vi "Initialize-object.vi"(7 "Heartbeat interval":dbl, 8 "error in (no error)":errorcluster, 9 "Client channel":refnum<queue>, 10 "Server channel":refnum<queue>) -> (0 "error out":errorcluster, 3 "Reference out":T1)   [LabVIEW 2013, in "CameraVision.lvlib" / "CV-Client.lvclass"]
doc: "Initialize the client resources and create a reference to the client object.\n\nRequires initialized communication channels (message queues), one for incoming (client) communication and one for outgoing (server) communication. These are generally intitialized by the 'server' instance which calls the main client vi."
uses:
  CV-Client.lvclass
  Object-reference.ctl
  SA-SLMAPI/Sources/Message.lvclass
  CV-Client.lvclass/CV-Client.ctl
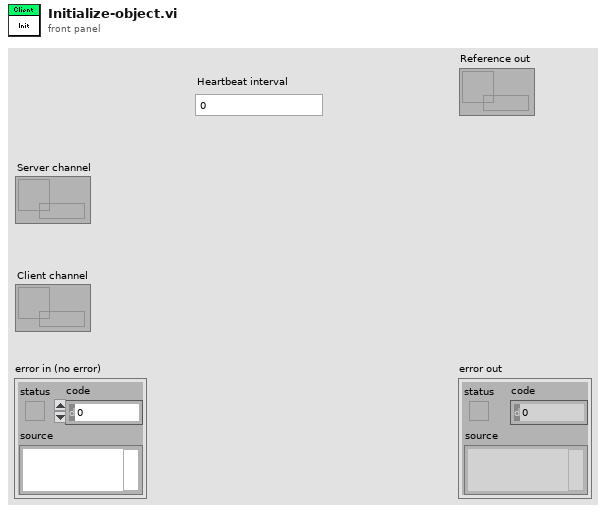
[diagram p1: front panel]
types:
  T1 = typedef "CameraVision.lvlib/CV-Client.lvclass/Object-reference.ctl" = refnum<data-value>
  T2 = typedef "CameraVision.lvlib/CV-Client.lvclass/Supported-modules.ctl" = enum16{"Server", "All", "SLMControl", "PowderDeposition", "StrategyParser", "CameraVision", "MaterialCharacterization", "StatusMonitor", "SLMSimulation", "LaserCharacterization"}
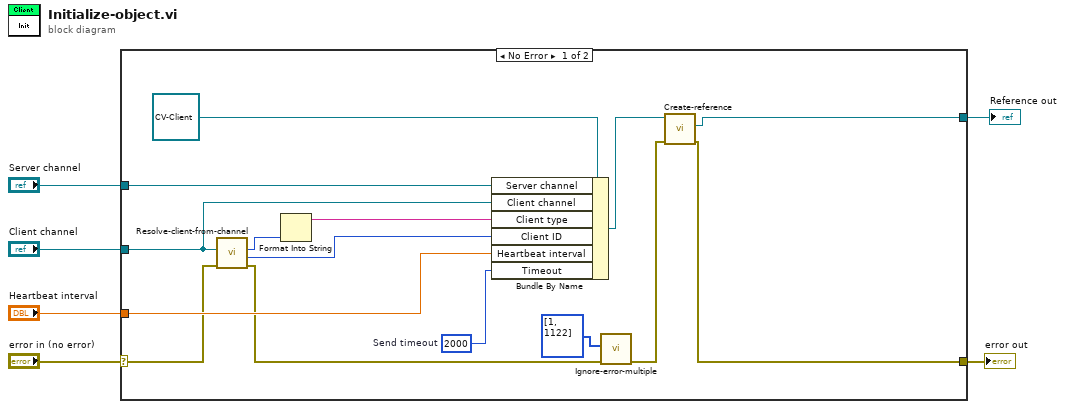
[diagram p0: block diagram]
diagram:
  n1 = case shown="No Error" "error in (no error)" {
    selector: "error in (no error)" -> [w13 w22]
    tunnel: [w21 w22] -> w5
    tunnel: [w20 _] -> w4
    tunnel: "Heartbeat interval" -> [w19 _]
    tunnel: "Client channel" -> [w14 _]
    tunnel: "Server channel" -> [w18 _]
    frame No Error {
      w15 = 2000  # Send timeout
      n2 = call "Resolve-client-from-channel.vi"("error in (no error)"=w13, "Client channel"=w14) -> ("error out"=w8:errorcluster, "Client ID"=w12:i32, "Client type"=w11:T2)  [unwired: 7 in]
      n3 = Format Into String(w11) -> (resulting string=w10:string)  [unwired: 3 in, 1 out]
      n4 = Bundle By Name(cluster=refnum<class "CV-Client.lvclass"> refnum ("Panes.lvclass"), "Server channel"=w18, "Client channel"=w14, "Client type"=w10, "Client ID"=w12, "Heartbeat interval"=w19, "Timeout"=w15) -> (w16:refnum<class "CV-Client.lvclass">)
      n5 = call "Ignore-error-multiple.vi"("error in (no error)"=w8, "Errors to ignore (1)"=i32[] [1, 1122]) -> ("error out"=w7:errorcluster)  [unwired: 9 in]
      n6 = call "Create-reference.vi"("error in (no error)"=w7, "Object in"=w16) -> ("error out"=w21:errorcluster, "Object reference"=w20:T1)  [unwired: 7 in, 1 out]
    }
    frame Error {
    }
  }
  "error out" <- w5
  "Reference out" <- w4
